vi "Build table output.vi"(8 "serialized text":string, 9 "BlueSerializer in":refnum<class "BlueSerializer.lvclass">, 10 "deserialized variant":variant, 11 "variant to data error":errorcluster) -> (3 "table output":string[](array[string]))   [LabVIEW 2019, in "Sports Unit Tests.lvclass"]
uses:
  Sports Unit Tests.lvclass
  <userlib>/Blue Origin/BlueSerialization/BlueSerializer/BlueSerializer.lvclass
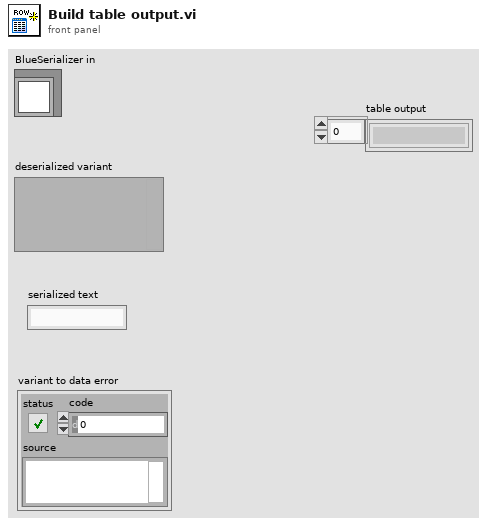
[diagram p1: front panel]
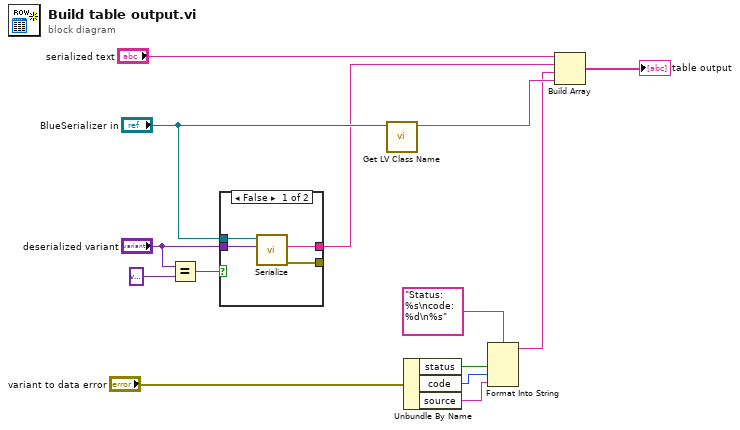
[diagram p0: block diagram]
diagram:
  n1 = Equal?(x="deserialized variant", y=variant) -> (x = y?=w1:bool)
  n2 = case shown="False" w1 {
    tunnel: "BlueSerializer in" -> [w18 _]
    tunnel: [w17 _] -> w11
    tunnel: [w16 _] -> _
    tunnel: "deserialized variant" -> [w15 _]
    frame False {
      n3 = call-dynamic "Serialize.vi"("Anything"=w15, "BlueSerializer in"=w18) -> ("error out"=w16:errorcluster, "Serialized Data"=w17:string)  [unwired: 7 in, 1 out]
    }
    frame True {
    }
  }
  n4 = call <vilib>:"Get LV Class Name.vi"("object"="BlueSerializer in") -> ("class name"=w13:string)  [unwired: 9 in, 1 out]
  n5 = Unbundle By Name("variant to data error") -> ("status"=w10:bool, "code"=w9:i32, "source"=w8:string)
  n6 = Format Into String(format string="Status: %s\ncode: %d\n%s", w10, w9, w8) -> (resulting string=w5:string)  [unwired: 2 in, 1 out]
  n7 = Build Array("serialized text", w11, w5, w13) -> (→"table output":string[])
